vi "Main.vi"() -> ()   [LabVIEW 2017]
uses:
  CTRLS/ListenMsg.ctl
  CTRLS/EventCluster.ctl
  CTRLS/MainCluster.ctl
  MainMsg.ctl
  CTRLS/DAQCluster.ctl
  DaqMsg.ctl
  CTRLS/GUICluster.ctl
  CTRLS/GUIMsg.ctl
  Keithley 2600 Series/Public/Channel.ctl
  <vilib>/Utility/file.llb/Write Delimited Spreadsheet (DBL).vi
  Keithley 2600 Series/Keithley 2600 Series.lvlib
panel:
  in  "b":dbl
  in  "a":dbl
  in  "?":enum32{"Diagram", "Air Pressure", "Efficiency"}(tab)
  out "Air flow, g/s":dbl format="%#_3g"
  out "Air press.(A), bar":dbl format="%#_3g"
  out "Water flow, m3/h":dbl format="%#_3g"
  out "Water press.(B), bar":dbl format="%#_3g"
  out "Nozzle force":dbl format="%#_3g"
  out "Water temp.":dbl format="%#_3g"
  out "Air Pressure Chart":dbl(graph)
  in  "Numeric 3":dbl
  in  "Numeric 2":dbl
  in  "Numeric":dbl
  out "Efficiency Chart":dbl(graph)
  in  "Keithley VISA name":refnum<visa-resource-name>="GPIB0::26::INSTR"
  out "SaveLED":bool
  out "MonLED":bool
  in  "clear error":bool
  out "error out":errorcluster
  in  "ForceChannel":refnum<k21>="TC_AI1"
  in  "WaterPchannel":refnum<k21>="TC_AI1"
  in  "AirPchannel":refnum<k21>="TC_AI1"
  in  "WaterFchannel":refnum<k21>="TC_AI1"
  in  "AirFchannel":refnum<k21>="TC_AI1"
  in  "WaterTchannel":refnum<k21>="TC_AI1"
  in  "Path to file":path=path "C:/Temp_save.txt"
  in  "Exit":bool
  in  "Save":bool
  in  "Monitoring":bool
  # "F = a* mV + b"
  # "Nozzle monitor. 2021. Michael Shustov. Excitonics"
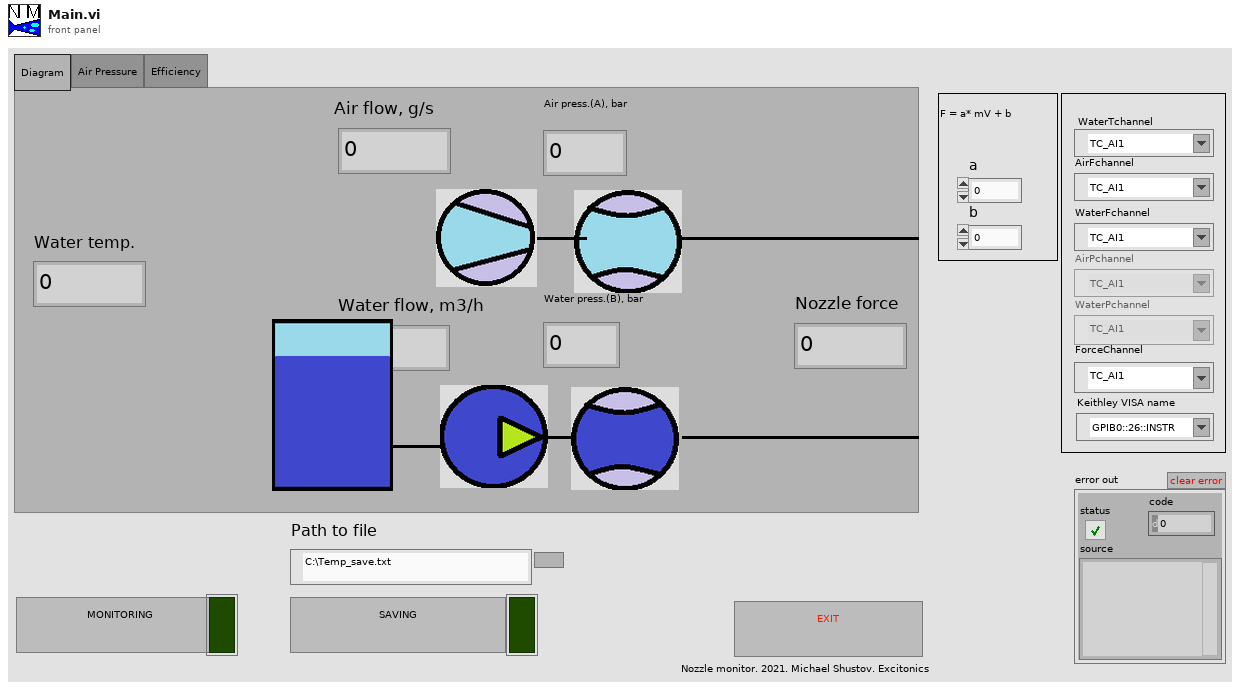
[diagram p1: front panel]
types:
  T1 = cluster{"Event out":refnum<queue>, "Main out":refnum<queue>, "DAC out":refnum<queue>, "GUI out":refnum<queue>}
  T2 = cluster{"WaterPchannel":refnum<vi>, "AirFchannel":refnum<vi>, "WaterFchannel":refnum<vi>, "AirPchannel":refnum<vi>, "ForceChannel":refnum<vi>, "WaterTchannel":refnum<vi>, "Water flow, m3/h":refnum<vi>, "Water press.(B), bar":refnum<vi>, "Water temp.":refnum<vi>, "Nozzle force":refnum<vi>, "Air press.(A), bar":refnum<vi>, "Monitoring":refnum<vi>, "Save":refnum<vi>, "Exit":refnum<vi>, "Path to file":refnum<vi>, "clear error":refnum<vi>, "error out":refnum<vi>, "Air flow, g/s":refnum<vi>, "MonLED":refnum<vi>, "SaveLED":refnum<vi>, "Keithley VISA name":refnum<vi>, "Air Pressure Chart":refnum<vi>, "a":refnum<vi>, "b":refnum<vi>, "Efficiency Chart":refnum<vi>}
  T3 = typedef "EventCluster.ctl" = cluster{"EventMsg":T4, "EventNum":dbl, "EventStr":string}
  T4 = typedef "ListenMsg.ctl" = enum16{"Init", "Halt", "Listen", "Error"}
  T5 = typedef "MainCluster.ctl" = cluster{"MainMsg":T6, "MainNum":dbl, "MainStr":string}
  T6 = typedef "MainMsg.ctl" = enum16{"Init", "Halt", "MonitorState", "SaveState", "Filename", "AirFlow", "WaterFlow", "AirPress", "WaterPress", "WaterTemp", "NozzleForce", "SaveAll", "Error", "Supervisor"}
  T7 = typedef "GUICluster.ctl" = cluster{"GUIMsg":T8, "GUINum":dbl, "GUIStr":string}
  T8 = typedef "GUIMsg.ctl" = enum16{"Init", "Halt", "WaterFlow", "AirFlow", "WaterPress", "AirPress", "WaterTemp", "NozzleForce", "SaveState", "MonState"}
  T9 = typedef "DAQCluster.ctl" = cluster{"DAQMsg":T10, "DAQNum":dbl, "DAQStr":string}
  T10 = typedef "DaqMsg.ctl" = enum16{"Init", "Halt", "GetMeasurement", "Stop", "Error"}
  T11 = cluster{"Temper":dbl, "AirFlow":dbl, "WaterFlow":dbl, "AirPressure":dbl, "WaterPressure":dbl, "Force":dbl, "Time":dbl}[]
  T12 = cluster{"Temper":dbl, "AirFlow":dbl, "WaterFlow":dbl, "AirPressure":dbl, "WaterPressure":dbl, "Force":dbl, "Time":dbl}
  T13 = typedef "Keithley 2600 Series.lvlib/Channel.ctl" = enum32{"Channel A", "Channel B"}
  T14 = enum32{"Current", "Voltage", "IV", "Resistance", "Power"}
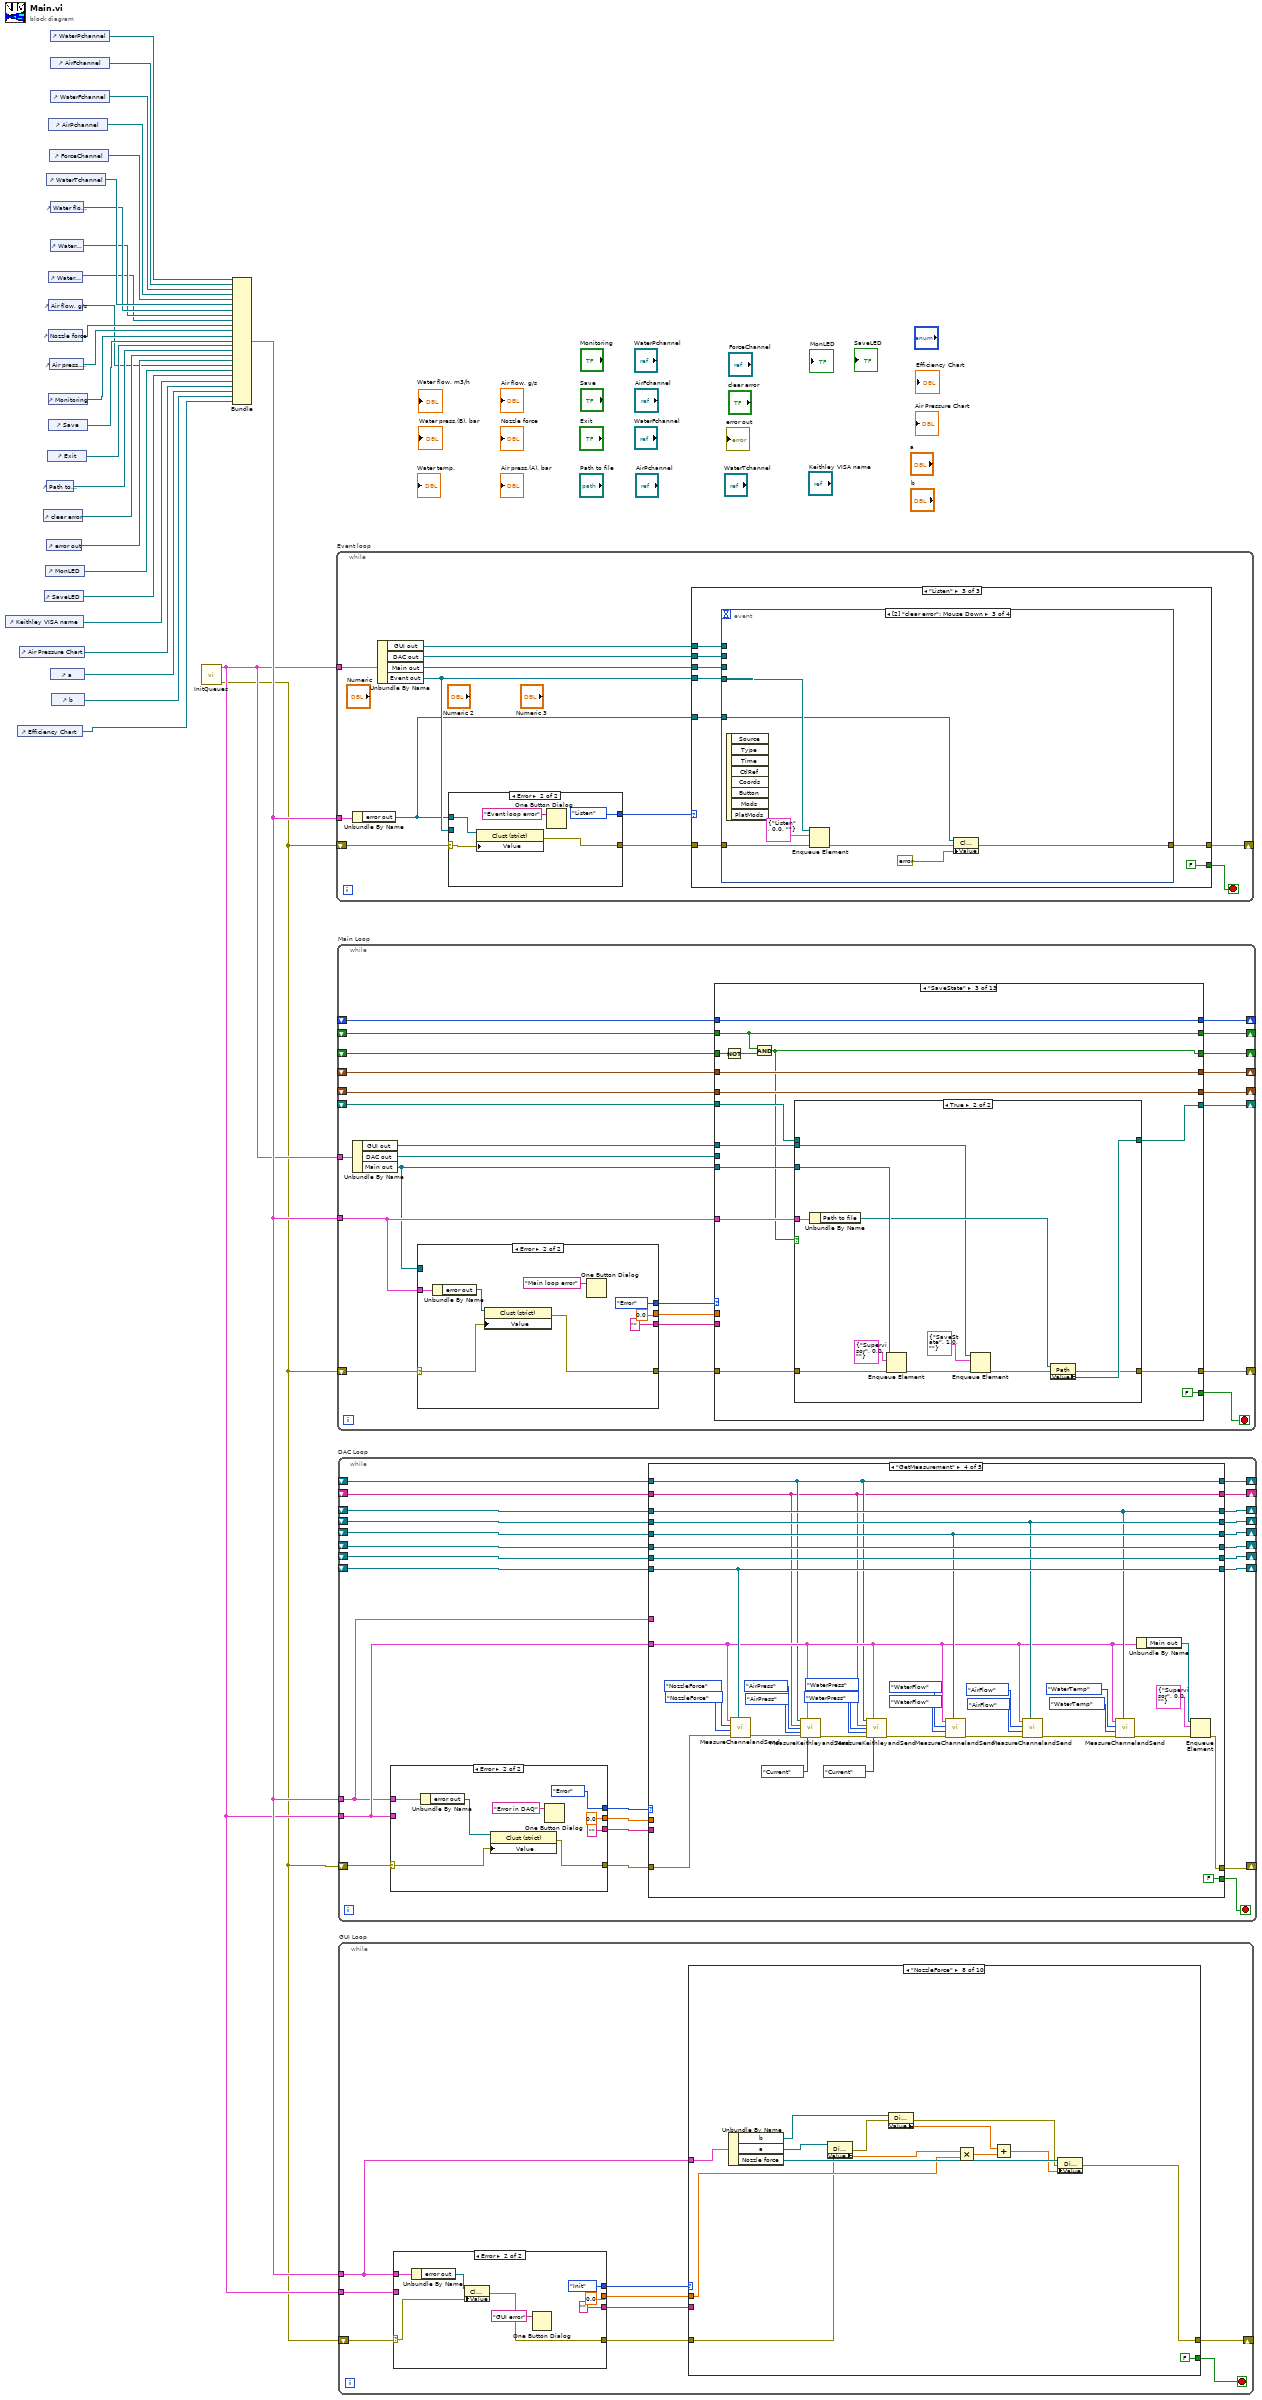
[diagram p0: block diagram]
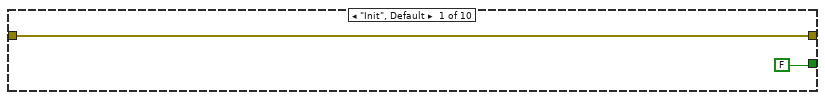
[diagram p2: hidden frame]
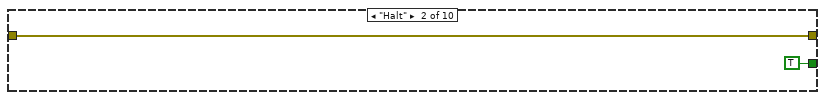
[diagram p3: hidden frame]
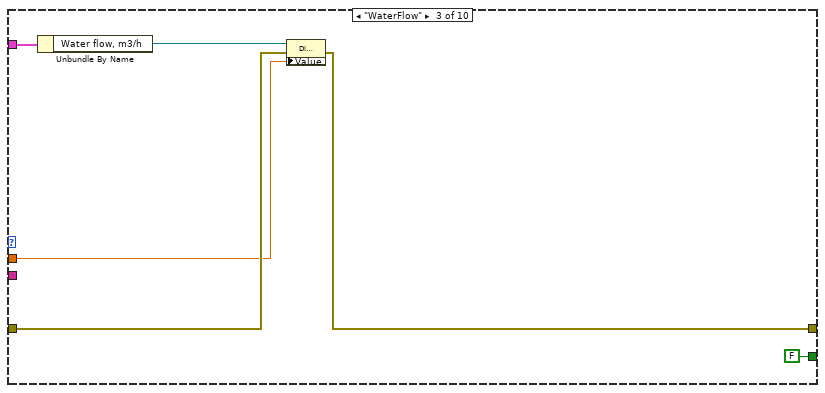
[diagram p4: hidden frame]
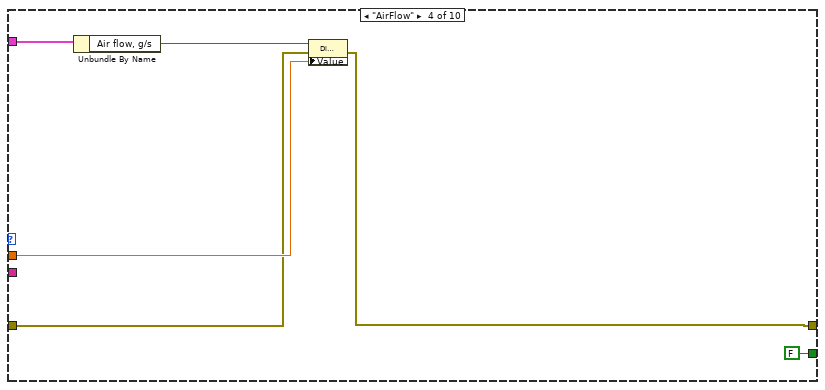
[diagram p5: hidden frame]
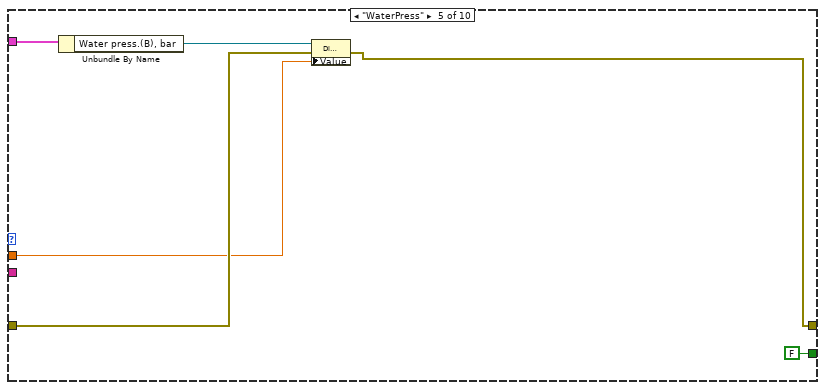
[diagram p6: hidden frame]
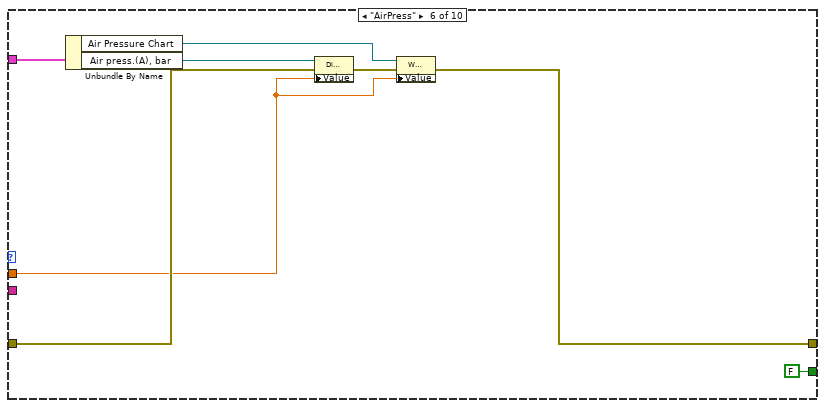
[diagram p7: hidden frame]
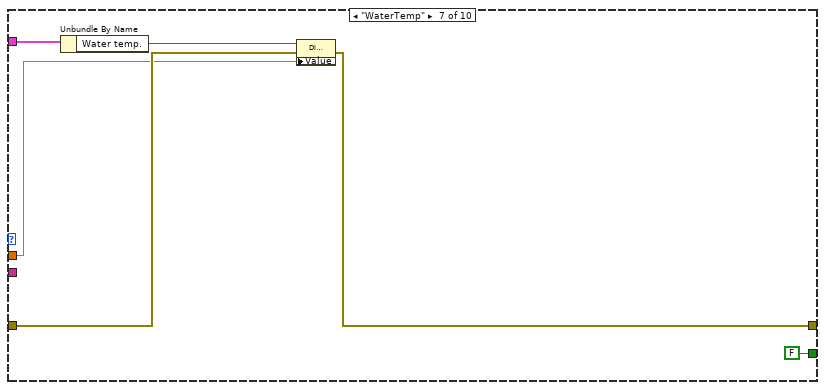
[diagram p8: hidden frame]
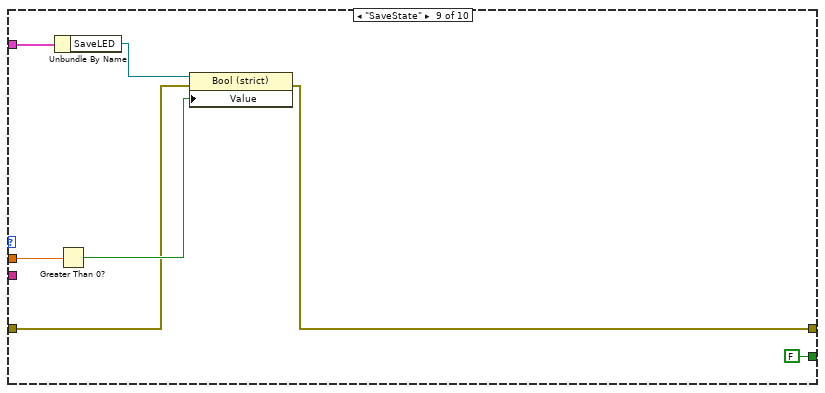
[diagram p9: hidden frame]
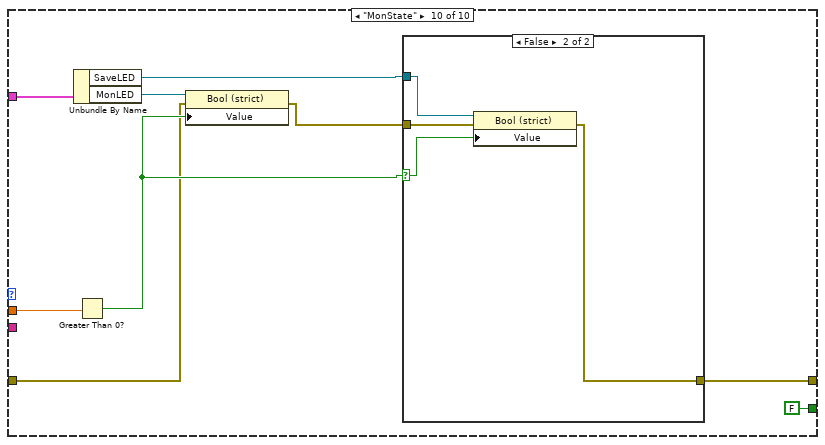
[diagram p10: hidden frame]
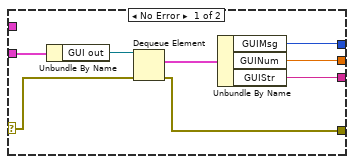
[diagram p12: hidden frame]
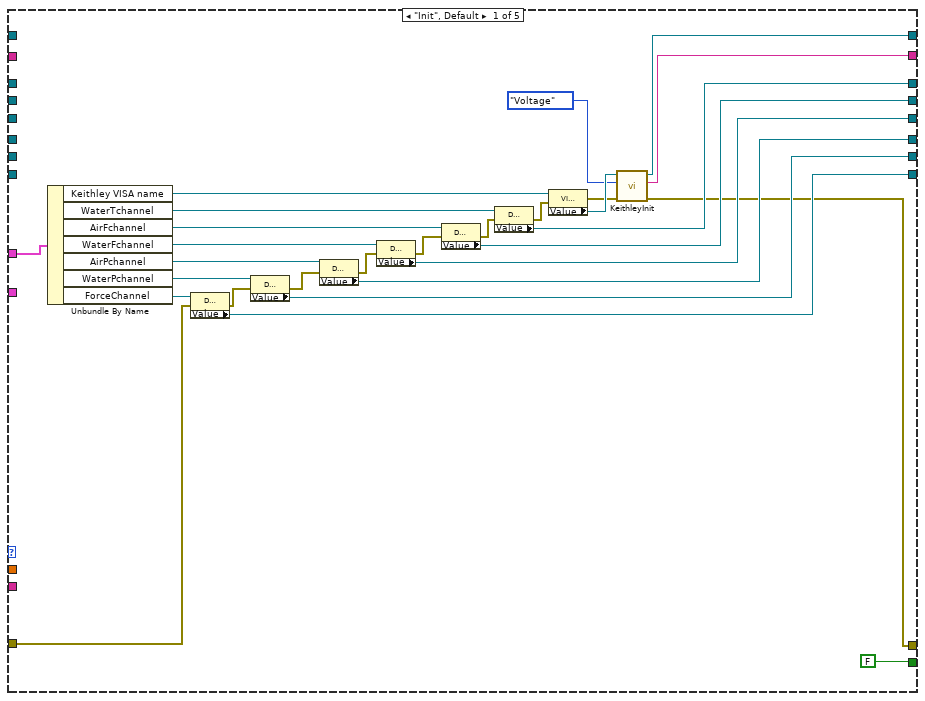
[diagram p13: hidden frame]
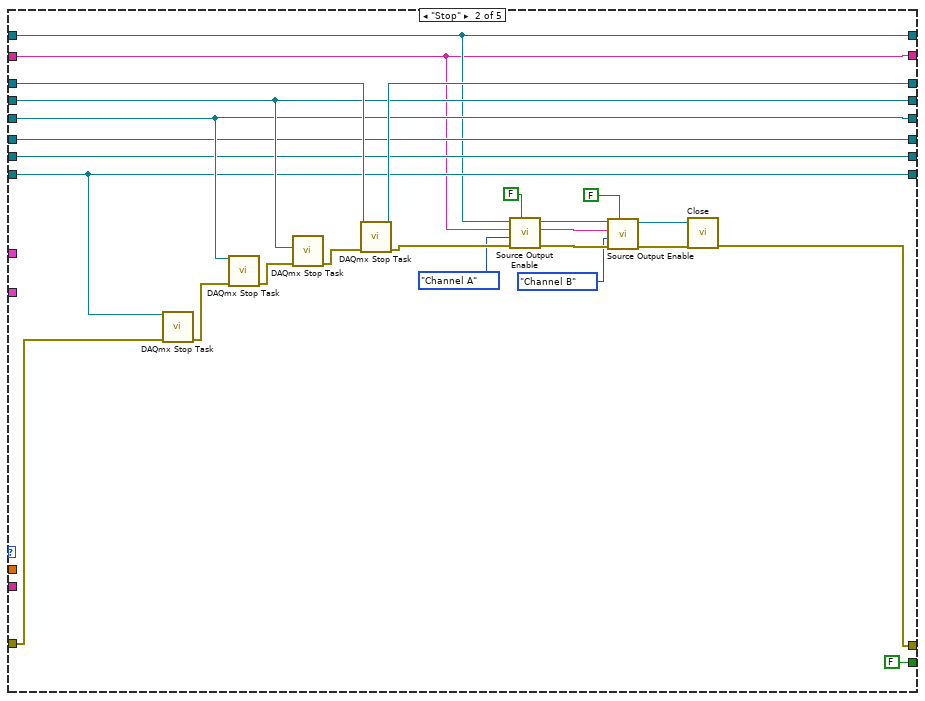
[diagram p14: hidden frame]
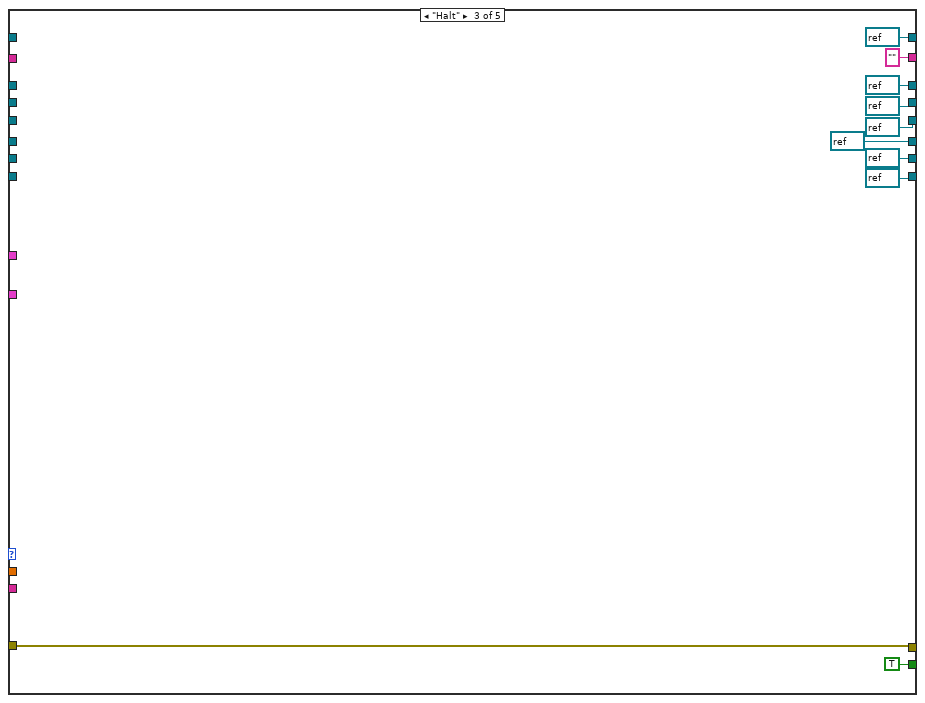
[diagram p15: hidden frame]
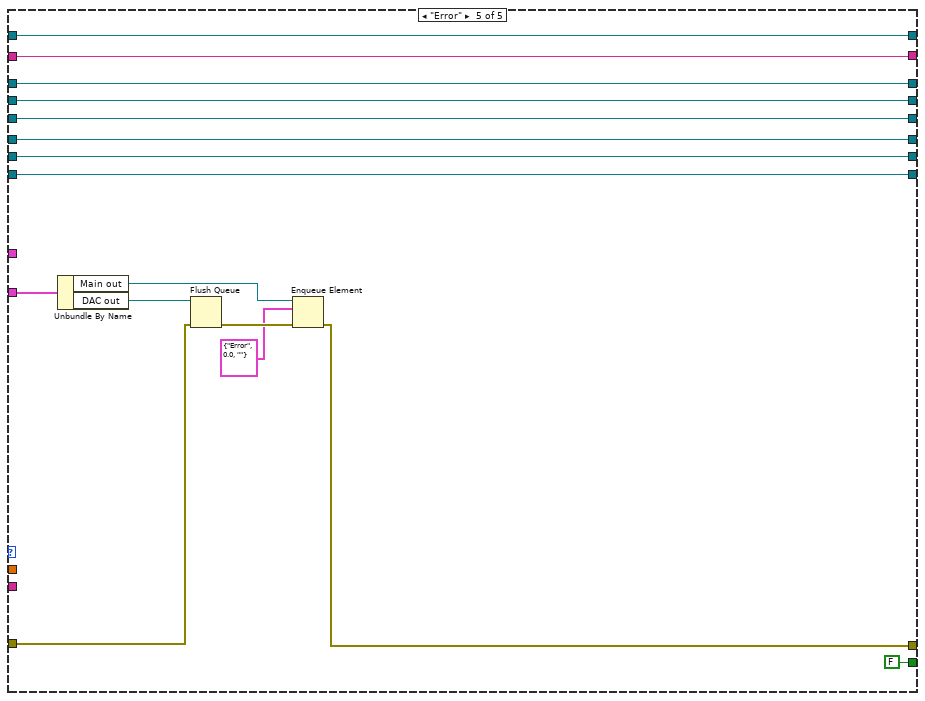
[diagram p16: hidden frame]
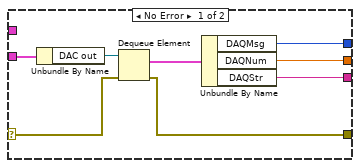
[diagram p17: hidden frame]
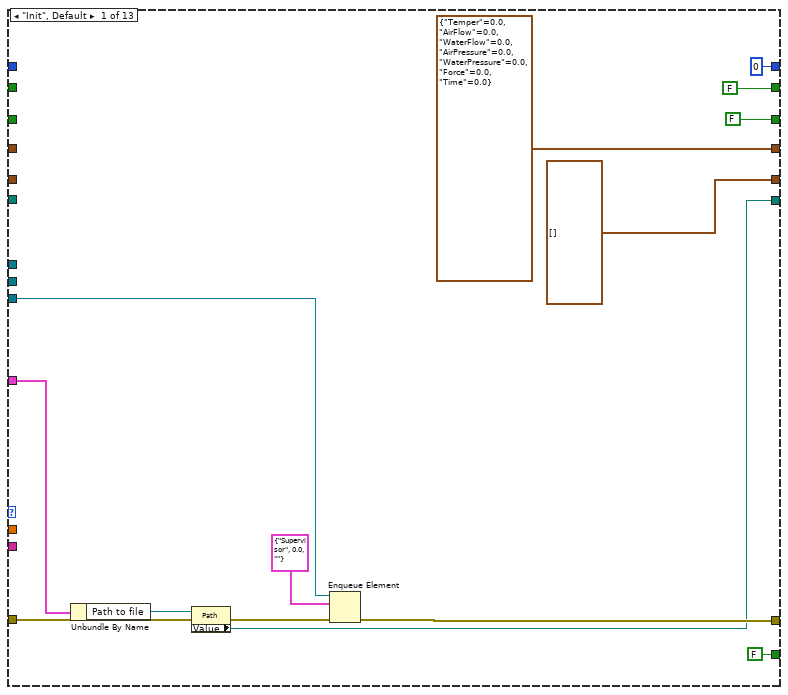
[diagram p18: hidden frame]
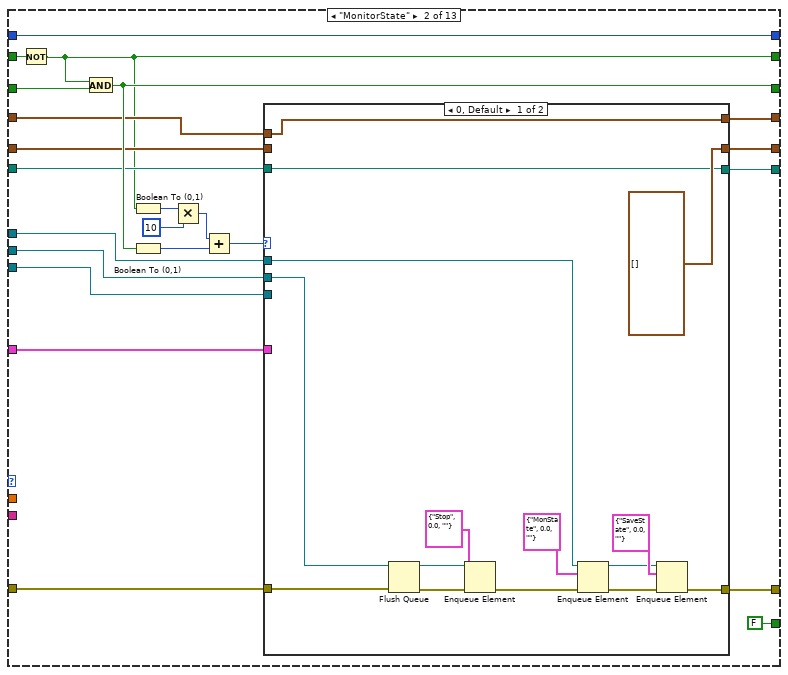
[diagram p19: hidden frame]
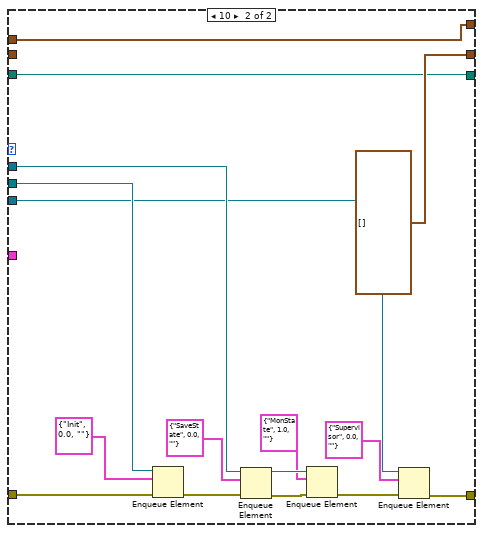
[diagram p20: hidden frame]
diagram:
  n1 = control-ref of="Keithley VISA name"() -> (w5:refnum<vi>)
  n2 = control-ref of="Efficiency Chart"() -> (w1:refnum<vi>)
  n3 = control-ref of="Air Pressure Chart"() -> (w4:refnum<vi>)
  n4 = control-ref of="clear error"() -> (w13:refnum<vi>)
  n5 = control-ref of="SaveLED"() -> (w6:refnum<vi>)
  n6 = control-ref of="MonLED"() -> (w7:refnum<vi>)
  n7 = control-ref of="Path to file"() -> (w14:refnum<vi>)
  n8 = control-ref of="WaterTchannel"() -> (w23:refnum<vi>)
  n9 = control-ref of="error out"() -> (w12:refnum<vi>)
  n10 = control-ref of="Exit"() -> (w15:refnum<vi>)
  n11 = control-ref of="AirPchannel"() -> (w25:refnum<vi>)
  n12 = control-ref of="Water temp."() -> (w20:refnum<vi>)
  n13 = control-ref of="Air flow, g/s"() -> (w11:refnum<vi>)
  n14 = control-ref of="Nozzle force"() -> (w19:refnum<vi>)
  n15 = control-ref of="Monitoring"() -> (w17:refnum<vi>)
  n16 = control-ref of="Save"() -> (w16:refnum<vi>)
  n17 = control-ref of="ForceChannel"() -> (w24:refnum<vi>)
  n18 = control-ref of="Air press.(A), bar"() -> (w18:refnum<vi>)
  n19 = control-ref of="Water flow, m3/h"() -> (w22:refnum<vi>)
  n20 = control-ref of="Water press.(B), bar"() -> (w21:refnum<vi>)
  n21 = control-ref of="WaterPchannel"() -> (w28:refnum<vi>)
  n22 = control-ref of="AirFchannel"() -> (w27:refnum<vi>)
  n23 = control-ref of="WaterFchannel"() -> (w26:refnum<vi>)
  n24 = control-ref of="a"() -> (w3:refnum<vi>)
  n25 = control-ref of="b"() -> (w2:refnum<vi>)
  n26 = call "InitQueues.vi"() -> ("error out"=w8:errorcluster, "QueueCluster"=w9:T1)  [unwired: 10 in]
  n27 = Bundle("WaterPchannel"=w28, "AirFchannel"=w27, "WaterFchannel"=w26, "AirPchannel"=w25, "ForceChannel"=w24, "WaterTchannel"=w23, "Water flow, m3/h"=w22, "Water press.(B), bar"=w21, "Water temp."=w20, "Nozzle force"=w19, "Air press.(A), bar"=w18, "Monitoring"=w17, "Save"=w16, "Exit"=w15, "Path to file"=w14, "clear error"=w13, "error out"=w12, "Air flow, g/s"=w11, "MonLED"=w7, "SaveLED"=w6, "Keithley VISA name"=w5, "Air Pressure Chart"=w4, "a"=w3, "b"=w2, "Efficiency Chart"=w1) -> (w10:T2)  [unwired: 1 in]
  n28 = while "Event loop" {
    tunnel: w10 -> [w37]
    shift-right: [w36] -> _
    shift-left: w8 -> [w40]
    tunnel: w9 -> [w35]
    stop <- w30 stop-if-true
    n29 = Unbundle By Name(w37) -> ("error out"=w31:refnum<vi>)
    n30 = Unbundle By Name(w35) -> ("GUI out"=w29:refnum<queue>, "DAC out"=w32:refnum<queue>, "Main out"=w34:refnum<queue>, "Event out"=w33:refnum<queue>)
    n31 = case shown="Error" w40 {
      selector: w40 -> [w95 w98]
      tunnel: [w93 ListenMsg."Listen" ("EventMsg")] -> w39
      tunnel: [w92 w97] -> w38
      tunnel: w31 -> [_ w99]
      tunnel: w33 -> [w91 _]
      frame No Error {
        n32 = Dequeue Element(queue=w91, error in (no error)=w95) -> (element=w94:T3, error out=w92:errorcluster)  [unwired: 1 in, 2 out]
        n33 = Unbundle(w94) -> ("EventMsg"=w93:T4)  [unwired: 2 out]
      }
      frame Error {
        n34 = property class="Clust (strict)"(reference=w99, "Value"=w98) -> (error out=w97:errorcluster)  [unwired: 1 in, 1 out]
        n35 = One Button Dialog(message="Event loop error") -> ()  [unwired: 1 in, 1 out]
      }
    }
    n36 = case shown="\"Listen\"" w39 {
      tunnel: w38 -> [w45 _ w56]
      tunnel: [w44 w47 w53] -> w36
      tunnel: w34 -> [_ _ w55]
      tunnel: w33 -> [w42 w48 w54]
      tunnel: w32 -> [_ _ w52]
      tunnel: w31 -> [_ _ w51]
      tunnel: [FALSE TRUE FALSE] -> w30
      tunnel: w29 -> [_ _ w49]
      frame "Init", Default {
        n37 = Enqueue Element(queue=w42, element=T3 {"EventMsg"=enum."Listen", "EventNum"=0.0, "EventStr"=""}, error in (no error)=w45) -> (error out=w44:errorcluster)  [unwired: 1 in, 2 out]
      }
      frame "Halt" {
        n38 = Flush Queue(queue=w48) -> (error out=w47:errorcluster)  [unwired: 1 in, 2 out]
      }
      frame "Listen" {
        n39 = event shown="[2] \"clear error\": Mouse Down" {
          selector: _ -> [_ _ _ _]
          dyn-events: _ -> [_ _ _ _]
          timeout: _ -> [_ _ _ _]
          tunnel: w56 -> [w63 w76 w82 w87]
          tunnel: w55 -> [w61 w73 _ w88]
          tunnel: w54 -> [w62 w75 w83 w89]
          tunnel: [w59 w64 w78 w86] -> w53
          tunnel: w52 -> [_ w71 _ _]
          tunnel: w51 -> [_ _ w81 _]
          tunnel: w49 -> [_ w70 _ _]
          event "Monitoring": Mouse Down {
            n40 = event-data() -> ()  [unwired: 1 in, 8 out]
            n41 = Enqueue Element(queue=w62, element=T3 {"EventMsg"=enum."Listen", "EventNum"=0.0, "EventStr"=""}, error in (no error)=w63) -> (error out=w60:errorcluster)  [unwired: 1 in, 2 out]
            n42 = Enqueue Element(queue=w61, element=T5 {"MainMsg"=enum."MonitorState", "MainNum"=0.0, "MainStr"=""}, error in (no error)=w60) -> (error out=w59:errorcluster)  [unwired: 1 in, 2 out]
          }
          event "Exit": Value Change {
            n43 = event-data() -> ()  [unwired: 1 in, 6 out]
            n44 = Enqueue Element(queue=w75, element=T3 {"EventMsg"=enum."Halt", "EventNum"=0.0, "EventStr"=""}, error in (no error)=w76) -> (error out=w74:errorcluster)  [unwired: 1 in, 2 out]
            n45 = Enqueue Element(queue=w73, element=T5 {"MainMsg"=enum."Halt", "MainNum"=0.0, "MainStr"=""}, error in (no error)=w74) -> (error out=w72:errorcluster)  [unwired: 1 in, 2 out]
            n46 = Enqueue Element(queue=w71, element=T9 {"DAQMsg"=enum."Halt", "DAQNum"=0.0, "DAQStr"=""}, error in (no error)=w72) -> (error out=w66:errorcluster)  [unwired: 1 in, 2 out]
            n47 = Enqueue Element(queue=w70, element=T7 {"GUIMsg"=enum."Halt", "GUINum"=0.0, "GUIStr"=""}, error in (no error)=w66) -> (error out=w64:errorcluster)  [unwired: 1 in, 2 out]
          }
          event "clear error": Mouse Down {
            n48 = event-data() -> ()  [unwired: 1 in, 8 out]
            n49 = Enqueue Element(queue=w83, element=T3 {"EventMsg"=enum."Listen", "EventNum"=0.0, "EventStr"=""}, error in (no error)=w82) -> (error out=w79:errorcluster)  [unwired: 1 in, 2 out]
            n50 = property class="Clust (strict)"(reference=w81, error in=w79, "Value"=errorcluster {"status"=FALSE, "code"=0, "source"=""}) -> (error out=w78:errorcluster)  [unwired: 1 out]
          }
          event "Save": Mouse Down {
            n51 = event-data() -> ()  [unwired: 1 in, 8 out]
            n52 = Enqueue Element(queue=w89, element=T3 {"EventMsg"=enum."Listen", "EventNum"=0.0, "EventStr"=""}, error in (no error)=w87) -> (error out=w90:errorcluster)  [unwired: 1 in, 2 out]
            n53 = Enqueue Element(queue=w88, element=T5 {"MainMsg"=enum."SaveState", "MainNum"=0.0, "MainStr"=""}, error in (no error)=w90) -> (error out=w86:errorcluster)  [unwired: 1 in, 2 out]
          }
        }
      }
    }
  }
  n54 = while "Main Loop" {
    tunnel: w10 -> [w113]
    tunnel: w9 -> [w124]
    shift-right: [w121] -> _
    shift-left: w8 -> [w120]
    shift-right: [w116] -> _
    shift-left: _ -> [w119]
    shift-right: [w117] -> _
    shift-left: _ -> [w118]
    shift-right: [w115] -> _
    shift-left: _ -> [w114]
    shift-right: [w106] -> _
    shift-left: _ -> [w105]
    shift-right: [w103] -> _
    shift-left: _ -> [w104]
    shift-right: [w102] -> _
    shift-left: _ -> [w101]
    stop <- w122 stop-if-true
    n55 = Unbundle By Name(w124) -> ("GUI out"=w110:refnum<queue>, "DAC out"=w111:refnum<queue>, "Main out"=w112:refnum<queue>)
    n56 = case shown="Error" w120 {
      selector: w120 -> [w397 w404]
      tunnel: [w396 w402] -> w123
      tunnel: w113 -> [_ w405]
      tunnel: w112 -> [w395 _]
      tunnel: [w393 MainMsg."Error" ("MainMsg")] -> w109
      tunnel: [w392 0.0 ("MainNum")] -> w108
      tunnel: [w391 "" ("MainStr")] -> w107
      frame No Error {
        n57 = Dequeue Element(queue=w395, error in (no error)=w397) -> (element=w394:T5, error out=w396:errorcluster)  [unwired: 1 in, 2 out]
        n58 = Unbundle By Name(w394) -> ("MainMsg"=w393:T6, "MainNum"=w392:dbl, "MainStr"=w391:string)
      }
      frame Error {
        n59 = Unbundle By Name(w405) -> ("error out"=w403:refnum<vi>)
        n60 = property class="Clust (strict)"(reference=w403, "Value"=w404) -> (error out=w402:errorcluster)  [unwired: 1 in, 1 out]
        n61 = One Button Dialog(message="Main loop error") -> ()  [unwired: 1 in, 1 out]
      }
    }
    n62 = case shown="\"SaveState\"" w109 {
      tunnel: w123 -> [w127 w149 w204 w230 w240 w250 w260 w270 w280 w301 w315 w366 w383]
      tunnel: [FALSE FALSE FALSE FALSE FALSE FALSE FALSE FALSE FALSE FALSE FALSE TRUE FALSE] -> w122
      tunnel: [w136 w151 w203 w230 w240 w250 w260 w270 w280 w287 w314 w368 w371] -> w121
      tunnel: w119 -> [_ w140 w194 w233 w242 w254 w263 w273 w283 w297 w325 w361 _]
      tunnel: w118 -> [_ w160 w197 w232 w241 w253 w262 w272 w282 w296 w324 w362 _]
      tunnel: [FALSE w155 w193 w232 w241 w253 w262 w272 w282 w296 w324 w362 FALSE] -> w117
      tunnel: [FALSE w139 w194 w233 w242 w254 w263 w273 w283 w297 w325 w361 FALSE] -> w116
      tunnel: [T12 {"Temper"=0.0, "AirFlow"=0.0, "WaterFlow"=0.0, "AirPressure"=0.0, "WaterPressure"=0.0, "Force"=0.0, "Time"=0.0} w142 w207 w235 w245 w255 w265 w275 w285 w295 w310 w363 T12 {"Temper"=0.0, "AirFlow"=0.0, "WaterFlow"=0.0, "AirPressure"=0.0, "WaterPressure"=0.0, "Force"=0.0, "Time"=0.0}] -> w115
      tunnel: w114 -> [_ w147 w207 w236 w246 w256 w266 w276 w286 w295 w311 w363 _]
      tunnel: w113 -> [w129 w146 w201 _ _ _ _ _ _ _ _ _ w374]
      tunnel: w112 -> [w134 w150 w205 _ _ _ _ _ _ w302 w316 w367 w389]
      tunnel: w111 -> [_ w153 _ _ _ _ _ _ _ _ w312 _ w388]
      tunnel: w110 -> [_ w152 w196 _ _ _ _ _ _ _ _ _ w382]
      tunnel: w108 -> [_ _ _ w231 w243 w251 w261 w271 w281 _ _ _ _]
      tunnel: w107 -> [_ _ _ _ _ _ _ _ _ _ _ _ _]
      tunnel: [0 w141 w198 w227 w237 w247 w257 w267 w278 w298 w318 w360 0] -> w106
      tunnel: w105 -> [_ w141 w198 w227 w237 w247 w257 w267 w278 w298 w317 w360 _]
      tunnel: w104 -> [_ w148 w202 w228 w238 w248 w258 w269 w279 w300 w308 w364 _]
      tunnel: [T11 [] ("appended array") w143 w202 w228 w238 w248 w258 w269 w279 T11 [] ("appended array") w307 w364 T11 [] ("appended array")] -> w103
      tunnel: [w126 w145 w200 w229 w239 w249 w259 w268 w277 w288 w309 w365 w373] -> w102
      tunnel: w101 -> [_ w144 w199 w229 w239 w249 w259 w268 w277 w292 w309 w365 _]
      frame "Init", Default {
        n63 = Unbundle By Name(w129) -> ("Path to file"=w128:refnum<vi>)
        n64 = property class="Path"(reference=w128, error in=w127) -> (error out=w125:errorcluster, "Value"=w126:path)  [unwired: 1 out]
        n65 = Enqueue Element(queue=w134, element=T5 {"MainMsg"=enum."Supervisor", "MainNum"=0.0, "MainStr"=""}, error in (no error)=w125) -> (error out=w136:errorcluster)  [unwired: 1 in, 2 out]
      }
      frame "MonitorState" {
        n66 = Not(x=w140) -> (.not. x?=w139:bool)
        n67 = And(x=w139, y=w160) -> (x .and. y?=w155:bool)
        n68 = Boolean To (0,1)(Boolean=w139) -> (0, 1=w159:i16)
        n69 = Boolean To (0,1)(Boolean=w155) -> (0, 1=w156:i16)
        n70 = Multiply(x=w159, y=i16 10) -> (x*y=w157:i16)
        n71 = Add(x=w157, y=w156) -> (x+y=w154:i16)
        n72 = case shown="0, Default" w154 {
          tunnel: w153 -> [w176 w192]
          tunnel: w152 -> [w171 w189]
          tunnel: [w172 w182] -> w151
          tunnel: w150 -> [_ w185]
          tunnel: w149 -> [w169 w190]
          tunnel: w148 -> [_ _]
          tunnel: w147 -> [w168 w183]
          tunnel: w146 -> [_ _]
          tunnel: [w167 w181] -> w145
          tunnel: w144 -> [w167 w181]
          tunnel: [T11 [] ("appended array") T11 [] ("appended array")] -> w143
          tunnel: [w168 w183] -> w142
          frame 0, Default {
            n73 = Flush Queue(queue=w176, error in (no error)=w169) -> (queue out=w165:refnum<queue>, error out=w164:errorcluster)  [unwired: 1 out]
            n74 = Enqueue Element(queue=w165, element=T9 {"DAQMsg"=enum."Stop", "DAQNum"=0.0, "DAQStr"=""}, error in (no error)=w164) -> (error out=w163:errorcluster)  [unwired: 1 in, 2 out]
            n75 = Enqueue Element(queue=w171, element=T7 {"GUIMsg"=enum."MonState", "GUINum"=0.0, "GUIStr"=""}, error in (no error)=w163) -> (queue out=w166:refnum<queue>, error out=w173:errorcluster)  [unwired: 1 in, 1 out]
            n76 = Enqueue Element(queue=w166, element=T7 {"GUIMsg"=enum."SaveState", "GUINum"=0.0, "GUIStr"=""}, error in (no error)=w173) -> (error out=w172:errorcluster)  [unwired: 1 in, 2 out]
          }
          frame 10 {
            n77 = Enqueue Element(queue=w192, element=T9 {"DAQMsg"=enum."Init", "DAQNum"=0.0, "DAQStr"=""}, error in (no error)=w190) -> (error out=w188:errorcluster)  [unwired: 1 in, 2 out]
            n78 = Enqueue Element(queue=w189, element=T7 {"GUIMsg"=enum."SaveState", "GUINum"=0.0, "GUIStr"=""}, error in (no error)=w188) -> (queue out=w178:refnum<queue>, error out=w179:errorcluster)  [unwired: 1 in, 1 out]
            n79 = Enqueue Element(queue=w178, element=T7 {"GUIMsg"=enum."MonState", "GUINum"=1.0, "GUIStr"=""}, error in (no error)=w179) -> (error out=w180:errorcluster)  [unwired: 1 in, 2 out]
            n80 = Enqueue Element(queue=w185, element=T5 {"MainMsg"=enum."Supervisor", "MainNum"=0.0, "MainStr"=""}, error in (no error)=w180) -> (error out=w182:errorcluster)  [unwired: 1 in, 2 out]
          }
        }
      }
      frame "SaveState" {
        n81 = Not(x=w197) -> (.not. x?=w195:bool)
        n82 = And(x=w194, y=w195) -> (x .and. y?=w193:bool)
        n83 = case shown="True" w193 {
          tunnel: w205 -> [w215 w226]
          tunnel: w204 -> [w213 w225]
          tunnel: [w208 w220] -> w203
          tunnel: w201 -> [_ w223]
          tunnel: [w212 w221] -> w200
          tunnel: w199 -> [w212 _]
          tunnel: w196 -> [w209 w217]
          frame False {
            n84 = Enqueue Element(queue=w215, element=T5 {"MainMsg"=enum."SaveAll", "MainNum"=0.0, "MainStr"=""}, error in (no error)=w213) -> (error out=w210:errorcluster)  [unwired: 1 in, 2 out]
            n85 = Enqueue Element(queue=w209, element=T7 {"GUIMsg"=enum."SaveState", "GUINum"=0.0, "GUIStr"=""}, error in (no error)=w210) -> (error out=w208:errorcluster)  [unwired: 1 in, 2 out]
          }
          frame True {
            n86 = Unbundle By Name(w223) -> ("Path to file"=w222:refnum<vi>)
            n87 = Enqueue Element(queue=w226, element=T5 {"MainMsg"=enum."Supervisor", "MainNum"=0.0, "MainStr"=""}, error in (no error)=w225) -> (error out=w218:errorcluster)  [unwired: 1 in, 2 out]
            n88 = Enqueue Element(queue=w217, element=T7 {"GUIMsg"=enum."SaveState", "GUINum"=1.0, "GUIStr"=""}, error in (no error)=w218) -> (error out=w219:errorcluster)  [unwired: 1 in, 2 out]
            n89 = property class="Path"(reference=w222, error in=w219) -> (error out=w220:errorcluster, "Value"=w221:path)  [unwired: 1 out]
          }
        }
      }
      frame "AirFlow" {
        n90 = Bundle By Name(cluster=w236, "AirFlow"=w231) -> (w235:T12)
      }
      frame "WaterFlow" {
        n91 = Bundle By Name(cluster=w246, "WaterFlow"=w243) -> (w245:T12)
      }
      frame "AirPress" {
        n92 = Bundle By Name(cluster=w256, "AirPressure"=w251) -> (w255:T12)
      }
      frame "WaterPress" {
        n93 = Bundle By Name(cluster=w266, "WaterPressure"=w261) -> (w265:T12)
      }
      frame "WaterTemp" {
        n94 = Bundle By Name(cluster=w276, "Temper"=w271) -> (w275:T12)
      }
      frame "NozzleForce" {
        n95 = Bundle By Name(cluster=w286, "Force"=w281) -> (w285:T12)
      }
      frame "SaveAll" {
        n96 = Enqueue Element(queue=w302, element=T5 {"MainMsg"=enum."Supervisor", "MainNum"=0.0, "MainStr"=""}, error in (no error)=w301) -> (error out=w293:errorcluster)  [unwired: 1 in, 2 out]
        n97 = for {
          tunnel: w300 -> [w306] mode=indexing
          tunnel: [w305] -> w290 mode=indexing
          tunnel: [w304] -> w291
          tunnel: w293 -> [w304]
          n98 = Cluster To Array(cluster=w306) -> (array=w305:dbl[])
        }
        n99 = call-poly <vilib>:"Write Delimited Spreadsheet.vi"("file path (dialog if empty)"=w292, "2D data"=w290, "append to file? (new file:F)"=TRUE, "error in (no error)"=w291) -> ("new file path (Not A Path if cancelled)"=w288:path, "error out"=w287:errorcluster)  [unwired: 10 in]
      }
      frame "Supervisor" {
        n100 = Boolean To (0,1)(Boolean=w324) -> (0, 1=w320:i16)
        n101 = Boolean To (0,1)(Boolean=w325) -> (0, 1=w323:i16)
        n102 = Multiply(x=w323, y=i16 10) -> (x*y=w321:i16)
        n103 = Add(x=w321, y=w320) -> (x+y=w319:i16)
        n104 = case shown="10" w319 {
          tunnel: [0 w331 w343] -> w318
          tunnel: w317 -> [_ w332 w340]
          tunnel: w316 -> [_ _ w342]
          tunnel: w315 -> [w326 w330 w339]
          tunnel: [w326 w329 w337] -> w314
          tunnel: w312 -> [_ w334 w341]
          frame 0, Default {
          }
          frame 10 {
            n105 = Increment(x=w332) -> (x+1=w331:i32)
            n106 = Enqueue Element(queue=w334, element=T9 {"DAQMsg"=enum."GetMeasurement", "DAQNum"=0.0, "DAQStr"=""}, error in (no error)=w330) -> (error out=w328:errorcluster)  [unwired: 1 in, 2 out]
            n107 = call "Time Delay"("error in (no error)"=w328, "Delay Time (s)"=0.1) -> ("error out"=w329:errorcluster)  [unwired: 9 in]
          }
          frame 11 {
            n108 = Greater?(x=w340, y=10) -> (0:w344:bool)
            n109 = case shown="False" w344 {
              tunnel: [w346 0] -> w343
              tunnel: w342 -> [_ w357]
              tunnel: w339 -> [w349 w356]
              tunnel: w341 -> [w350 w355]
              tunnel: [w348 w352] -> w338
              tunnel: w340 -> [w347 _]
              frame False {
                n110 = Increment(x=w347) -> (x+1=w346:i32)
                n111 = Enqueue Element(queue=w350, element=T9 {"DAQMsg"=enum."GetMeasurement", "DAQNum"=0.0, "DAQStr"=""}, error in (no error)=w349) -> (error out=w348:errorcluster)  [unwired: 1 in, 2 out]
              }
              frame True {
                n112 = Enqueue Element(queue=w357, element=T5 {"MainMsg"=enum."SaveAll", "MainNum"=0.0, "MainStr"=""}, error in (no error)=w356) -> (error out=w354:errorcluster)  [unwired: 1 in, 2 out]
                n113 = Enqueue Element(queue=w355, element=T9 {"DAQMsg"=enum."GetMeasurement", "DAQNum"=0.0, "DAQStr"=""}, error in (no error)=w354) -> (error out=w352:errorcluster)  [unwired: 1 in, 2 out]
              }
            }
            n114 = call "Time Delay2"("error in (no error)"=w338, "Delay Time (s)"=0.1) -> ("error out"=w337:errorcluster)  [unwired: 9 in]
          }
        }
        n115 = call "AddTimeToArr.vi"("Arr in"=w308, "Cluster in"=w311) -> ("Arr out"=w307:T11, "Cluster out"=w310:T12)  [unwired: 8 in]
      }
      frame "Halt" {
        n116 = Flush Queue(queue=w367, error in (no error)=w366) -> (error out=w368:errorcluster)  [unwired: 2 out]
      }
      frame "Error" {
        n117 = Flush Queue(queue=w389, error in (no error)=w383) -> (error out=w387:errorcluster)  [unwired: 2 out]
        n118 = Flush Queue(queue=w388, error in (no error)=w387) -> (error out=w370:errorcluster)  [unwired: 2 out]
        n119 = Enqueue Element(queue=w382, element=T7 {"GUIMsg"=enum."SaveState", "GUINum"=0.0, "GUIStr"=""}, error in (no error)=w370) -> (queue out=w380:refnum<queue>, error out=w379:errorcluster)  [unwired: 1 in, 1 out]
        n120 = Enqueue Element(queue=w380, element=T7 {"GUIMsg"=enum."MonState", "GUINum"=0.0, "GUIStr"=""}, error in (no error)=w379) -> (error out=w372:errorcluster)  [unwired: 1 in, 2 out]
        n121 = Unbundle By Name(w374) -> ("Path to file"=w375:refnum<vi>)
        n122 = property class="Path"(reference=w375, error in=w372) -> (error out=w371:errorcluster, "Value"=w373:path)  [unwired: 1 out]
      }
    }
  }
  n123 = while "DAC Loop" {
    tunnel: w10 -> [w410]
    tunnel: w9 -> [w412]
    shift-right: [w427] -> _
    shift-left: _ -> [w421]
    shift-right: [w426] -> _
    shift-left: _ -> [w420]
    shift-right: [w425] -> _
    shift-left: _ -> [w419]
    shift-right: [w424] -> _
    shift-left: _ -> [w418]
    shift-right: [w423] -> _
    shift-left: _ -> [w417]
    shift-right: [w422] -> _
    shift-left: _ -> [w416]
    shift-right: [w414] -> _
    shift-left: w8 -> [w413]
    shift-right: [w408] -> _
    shift-left: _ -> [w409]
    shift-right: [w407] -> _
    shift-left: _ -> [w406]
    stop <- w415 stop-if-true
    n124 = case shown="Error" w413 {
      selector: w413 -> [w551 w555]
      tunnel: [w549 w553] -> w430
      tunnel: [w548 DaqMsg."Error" ("DAQMsg")] -> w411
      tunnel: [w547 0.0 ("DAQNum")] -> w429
      tunnel: [w546 "" ("DAQStr")] -> w428
      tunnel: w412 -> [w544 _]
      tunnel: w410 -> [_ w556]
      frame No Error {
        n125 = Unbundle By Name(w544) -> ("DAC out"=w545:refnum<queue>)
        n126 = Dequeue Element(queue=w545, error in (no error)=w551) -> (element=w550:T9, error out=w549:errorcluster)  [unwired: 1 in, 2 out]
        n127 = Unbundle By Name(w550) -> ("DAQMsg"=w548:T10, "DAQNum"=w547:dbl, "DAQStr"=w546:string)
      }
      frame Error {
        n128 = Unbundle By Name(w556) -> ("error out"=w554:refnum<vi>)
        n129 = property class="Clust (strict)"(reference=w554, "Value"=w555) -> (error out=w553:errorcluster)  [unwired: 1 in, 1 out]
        n130 = One Button Dialog(message="Error in DAQ") -> ()  [unwired: 1 in, 1 out]
      }
    }
    n131 = case shown="\"GetMeasurement\"" w411 {
      tunnel: w430 -> [w457 w473 w486 w527 w532]
      tunnel: w429 -> [_ _ _ _ _]
      tunnel: w428 -> [_ _ _ _ _]
      tunnel: w410 -> [w458 _ _ _ _]
      tunnel: [w440 w476 refnum<k21> refnum ("Value") w523 w534] -> w423
      tunnel: [w441 w477 refnum<k21> refnum ("Value") w522 w535] -> w424
      tunnel: [w443 w479 refnum<k21> refnum ("Value") w515 w537] -> w426
      tunnel: [w442 w478 refnum<k21> refnum ("Value") w521 w536] -> w425
      tunnel: [w444 w480 refnum<k21> refnum ("Value") w511 w538] -> w427
      tunnel: [w439 w475 refnum<k21> refnum ("Value") w524 w533] -> w422
      tunnel: w421 -> [_ w483 _ w511 w538]
      tunnel: w420 -> [_ w479 _ w515 w537]
      tunnel: w419 -> [_ w478 _ w521 w536]
      tunnel: w418 -> [_ w477 _ w522 w535]
      tunnel: w417 -> [_ w476 _ w523 w534]
      tunnel: w416 -> [_ w475 _ w524 w533]
      tunnel: [FALSE FALSE TRUE FALSE FALSE] -> w415
      tunnel: [w433 w461 w486 w506 w531] -> w414
      tunnel: w412 -> [_ _ _ w498 w543]
      tunnel: w409 -> [_ w460 _ w495 w529]
      tunnel: [w432 w460 refnum<visa-resource-name> refnum ("VISA Refnum out") w495 w529] -> w408
      tunnel: [w431 w459 "" ("Node Out") w494 w528] -> w407
      tunnel: w406 -> [_ w459 _ w494 w528]
      frame "Init", Default {
        n132 = Unbundle By Name(w458) -> ("Keithley VISA name"=w437:refnum<vi>, "WaterTchannel"=w447:refnum<vi>, "AirFchannel"=w448:refnum<vi>, "WaterFchannel"=w450:refnum<vi>, "AirPchannel"=w452:refnum<vi>, "WaterPchannel"=w454:refnum<vi>, "ForceChannel"=w456:refnum<vi>)
        n133 = property class="DAQmxName (strict)"(reference=w456, error in=w457) -> (error out=w455:errorcluster, "Value"=w439:refnum<k21>)  [unwired: 1 out]
        n134 = property class="DAQmxName (strict)"(reference=w454, error in=w455) -> (error out=w453:errorcluster, "Value"=w440:refnum<k21>)  [unwired: 1 out]
        n135 = property class="DAQmxName (strict)"(reference=w452, error in=w453) -> (error out=w451:errorcluster, "Value"=w441:refnum<k21>)  [unwired: 1 out]
        n136 = property class="DAQmxName (strict)"(reference=w450, error in=w451) -> (error out=w449:errorcluster, "Value"=w442:refnum<k21>)  [unwired: 1 out]
        n137 = property class="DAQmxName (strict)"(reference=w448, error in=w449) -> (error out=w446:errorcluster, "Value"=w443:refnum<k21>)  [unwired: 1 out]
        n138 = property class="DAQmxName (strict)"(reference=w447, error in=w446) -> (error out=w438:errorcluster, "Value"=w444:refnum<k21>)  [unwired: 1 out]
        n139 = property class="VISAName"(reference=w437, error in=w438) -> (error out=w434:errorcluster, "Value"=w436:refnum<visa-resource-name>)  [unwired: 1 out]
        n140 = call "KeithleyInit.vi"("error in (no error)"=w434, "SourceFunction"=enum32{"Current", "Voltage"}."Voltage", "VISA Refnum in"=w436) -> ("error out"=w433:errorcluster, "Node Out"=w431:string, "VISA Refnum out"=w432:refnum<visa-resource-name>)  [unwired: 6 in]
      }
      frame "Stop" {
        n141 = call <vilib>:"DAQmx Stop Task.vi"("task/channels in"=w475, "error in"=w473) -> ("error out"=w471:errorcluster)  [unwired: 12 in, 1 out]
        n142 = call <vilib>:"DAQmx Stop Task.vi"("task/channels in"=w478, "error in"=w471) -> ("error out"=w482:errorcluster)  [unwired: 12 in, 1 out]
        n143 = call <vilib>:"DAQmx Stop Task.vi"("task/channels in"=w479, "error in"=w482) -> ("error out"=w481:errorcluster)  [unwired: 12 in, 1 out]
        n144 = call <vilib>:"DAQmx Stop Task.vi"("task/channels in"=w483, "error in"=w481) -> ("task out"=w480:refnum<k21>, "error out"=w470:errorcluster)  [unwired: 12 in]
        n145 = call "Source Output Enable.vi"("Output (Off)"=FALSE, "error in (no error)"=w470, "Channel (Channel A)"=Channel."Channel A", "Node In"=w459, "VISA resource name"=w460) -> ("error out"=w467:errorcluster, "Node Out"=w469:string, "VISA resource name out"=w468:refnum<visa-resource-name>)  [unwired: 4 out]
        n146 = call "Source Output Enable.vi"("Output (Off)"=FALSE, "error in (no error)"=w467, "Channel (Channel A)"=Channel."Channel B", "Node In"=w469, "VISA resource name"=w468) -> ("error out"=w464:errorcluster, "VISA resource name out"=w463:refnum<visa-resource-name>)  [unwired: 5 out]
        n147 = call "Close.vi"("error in (no error)"=w464, "VISA resource name"=w463) -> ("error out"=w461:errorcluster)  [unwired: 9 in]
      }
      frame "Halt" {
      }
      frame "GetMeasurement" {
        n148 = call "MeasureChannelandSend.vi"("DAQChannel"=w524, "error in (no error)"=w527, "GUIMsg"=GUIMsg."NozzleForce", "MainMsg"=MainMsg."NozzleForce", "QueueCluster"=w498) -> ("error out"=w503:errorcluster)  [unwired: 6 in]
        n149 = call "MeasureKeithleyandSend.vi"("Keithley Visa name"=w495, "QueueCluster"=w498, "Node In"=w494, "MainMsg"=MainMsg."AirPress", "GUIMsg"=GUIMsg."AirPress", "error in (no error)"=w503, "MeasureFunction"=T14."Current") -> ("error out"=w502:errorcluster)  [unwired: 8 in]
        n150 = call "MeasureKeithleyandSend.vi"("Keithley Visa name"=w495, "QueueCluster"=w498, "Node In"=w494, "MainMsg"=MainMsg."WaterPress", "GUIMsg"=GUIMsg."WaterPress", "error in (no error)"=w502, "MeasureFunction"=T14."Current") -> ("error out"=w501:errorcluster)  [unwired: 8 in]
        n151 = call "MeasureChannelandSend.vi"("DAQChannel"=w521, "error in (no error)"=w501, "GUIMsg"=GUIMsg."WaterFlow", "MainMsg"=MainMsg."WaterFlow", "QueueCluster"=w498) -> ("error out"=w516:errorcluster)  [unwired: 6 in]
        n152 = call "MeasureChannelandSend.vi"("DAQChannel"=w515, "error in (no error)"=w516, "GUIMsg"=GUIMsg."AirFlow", "MainMsg"=MainMsg."AirFlow", "QueueCluster"=w498) -> ("error out"=w513:errorcluster)  [unwired: 6 in]
        n153 = call "MeasureChannelandSend.vi"("DAQChannel"=w511, "error in (no error)"=w513, "GUIMsg"=GUIMsg."WaterTemp", "MainMsg"=MainMsg."WaterTemp", "QueueCluster"=w498) -> ("error out"=w509:errorcluster)  [unwired: 6 in]
        n154 = Unbundle By Name(w498) -> ("Main out"=w508:refnum<queue>)
        n155 = Enqueue Element(queue=w508, element=T5 {"MainMsg"=enum."Supervisor", "MainNum"=0.0, "MainStr"=""}, error in (no error)=w509) -> (error out=w506:errorcluster)  [unwired: 1 in, 2 out]
      }
      frame "Error" {
        n156 = Unbundle By Name(w543) -> ("Main out"=w541:refnum<queue>, "DAC out"=w542:refnum<queue>)
        n157 = Flush Queue(queue=w542, error in (no error)=w532) -> (error out=w540:errorcluster)  [unwired: 2 out]
        n158 = Enqueue Element(queue=w541, element=T5 {"MainMsg"=enum."Error", "MainNum"=0.0, "MainStr"=""}, error in (no error)=w540) -> (error out=w531:errorcluster)  [unwired: 1 in, 2 out]
      }
    }
  }
  n159 = while "GUI Loop" {
    tunnel: w10 -> [w560]
    tunnel: w9 -> [w568]
    shift-right: [w563] -> _
    shift-left: w8 -> [w562]
    stop <- w561 stop-if-true
    n160 = case shown="Error" w562 {
      selector: w562 -> [w645 w654]
      tunnel: w568 -> [w647 _]
      tunnel: [w643 GUIMsg."Init" ("GUIMsg")] -> w567
      tunnel: [w642 0.0 ("GUINum")] -> w564
      tunnel: [w641 "" ("GUIStr")] -> w565
      tunnel: [w640 w652] -> w566
      tunnel: w560 -> [_ w655]
      frame No Error {
        n161 = Unbundle By Name(w647) -> ("GUI out"=w646:refnum<queue>)
        n162 = Dequeue Element(queue=w646, error in (no error)=w645) -> (element=w644:T7, error out=w640:errorcluster)  [unwired: 1 in, 2 out]
        n163 = Unbundle By Name(w644) -> ("GUIMsg"=w643:T8, "GUINum"=w642:dbl, "GUIStr"=w641:string)
      }
      frame Error {
        n164 = Unbundle By Name(w655) -> ("error out"=w653:refnum<vi>)
        n165 = property class="Clust (strict)"(reference=w653, "Value"=w654) -> (error out=w652:errorcluster)  [unwired: 1 in, 1 out]
        n166 = One Button Dialog(message="GUI error") -> ()  [unwired: 1 in, 1 out]
      }
    }
    n167 = case shown="\"NozzleForce\"" w567 {
      tunnel: w566 -> [w570 w571 w576 w581 w588 w596 w602 w611 w620 w628]
      tunnel: w565 -> [_ _ _ _ _ _ _ _ _ _]
      tunnel: w564 -> [_ _ w574 w582 w587 w592 w601 w614 w625 w633]
      tunnel: [w570 w571 w573 w580 w586 w591 w600 w616 w619 w626] -> w563
      tunnel: [FALSE TRUE FALSE FALSE FALSE FALSE FALSE FALSE FALSE FALSE] -> w561
      tunnel: w560 -> [_ _ w577 w583 w589 w597 w603 w617 w624 w634]
      frame "Init", Default {
      }
      frame "Halt" {
      }
      frame "WaterFlow" {
        n168 = Unbundle By Name(w577) -> ("Water flow, m3/h"=w575:refnum<vi>)
        n169 = property class="DigNum (strict)"(reference=w575, error in=w576, "Value"=w574) -> (error out=w573:errorcluster)  [unwired: 1 out]
      }
      frame "AirFlow" {
        n170 = Unbundle By Name(w583) -> ("Air flow, g/s"=w584:refnum<vi>)
        n171 = property class="DigNum (strict)"(reference=w584, error in=w581, "Value"=w582) -> (error out=w580:errorcluster)  [unwired: 1 out]
      }
      frame "WaterPress" {
        n172 = Unbundle By Name(w589) -> ("Water press.(B), bar"=w590:refnum<vi>)
        n173 = property class="DigNum (strict)"(reference=w590, error in=w588, "Value"=w587) -> (error out=w586:errorcluster)  [unwired: 1 out]
      }
      frame "AirPress" {
        n174 = Unbundle By Name(w597) -> ("Air Pressure Chart"=w594:refnum<vi>, "Air press.(A), bar"=w598:refnum<vi>)
        n175 = property class="DigNum (strict)"(reference=w598, error in=w596, "Value"=w592) -> (error out=w593:errorcluster)  [unwired: 1 out]
        n176 = property class="WFChart (strict)"(reference=w594, error in=w593, "Value"=w592) -> (error out=w591:errorcluster)  [unwired: 1 out]
      }
      frame "WaterTemp" {
        n177 = Unbundle By Name(w603) -> ("Water temp."=w604:refnum<vi>)
        n178 = property class="DigNum (strict)"(reference=w604, error in=w602, "Value"=w601) -> (error out=w600:errorcluster)  [unwired: 1 out]
      }
      frame "NozzleForce" {
        n179 = Unbundle By Name(w617) -> ("b"=w612:refnum<vi>, "a"=w613:refnum<vi>, "Nozzle force"=w618:refnum<vi>)
        n180 = property class="DigNum (strict)"(reference=w613, error in=w611) -> (error out=w610:errorcluster, "Value"=w609:dbl)  [unwired: 1 out]
        n181 = property class="DigNum (strict)"(reference=w612, error in=w610) -> (error out=w606:errorcluster, "Value"=w608:dbl)  [unwired: 1 out]
        n182 = Multiply(x=w609, y=w614) -> (x*y=w607:dbl)
        n183 = Add(x=w608, y=w607) -> (x+y=w605:dbl)
        n184 = property class="DigNum (strict)"(reference=w618, error in=w606, "Value"=w605) -> (error out=w616:errorcluster)  [unwired: 1 out]
      }
      frame "SaveState" {
        n185 = Unbundle By Name(w624) -> ("SaveLED"=w622:refnum<vi>)
        n186 = Greater Than 0?(x=w625) -> (x > 0?=w621:bool)
        n187 = property class="Bool (strict)"(reference=w622, error in=w620, "Value"=w621) -> (error out=w619:errorcluster)  [unwired: 1 out]
      }
      frame "MonState" {
        n188 = Unbundle By Name(w634) -> ("SaveLED"=w629:refnum<vi>, "MonLED"=w631:refnum<vi>)
        n189 = Greater Than 0?(x=w633) -> (x > 0?=w630:bool)
        n190 = property class="Bool (strict)"(reference=w631, error in=w628, "Value"=w630) -> (error out=w627:errorcluster)  [unwired: 1 out]
        n191 = case shown="False" w630 {
          selector: w630 -> [_ w636]
          tunnel: w629 -> [_ w637]
          tunnel: w627 -> [w635 w639]
          tunnel: [w635 w638] -> w626
          frame True {
          }
          frame False {
            n192 = property class="Bool (strict)"(reference=w637, error in=w639, "Value"=w636) -> (error out=w638:errorcluster)  [unwired: 1 out]
          }
        }
      }
    }
  }
